vi "update_tab.vi"(8 "配置":T1 {"串口通信UI"."Format" items=["标准帧", "扩展帧"]; "串口通信UI"."Type" items=["数据帧", "远程帧"]; "串口通信UI"."ID" format="0x%x"; "串口通信UI"."Fliter" items=["接收所有类型"=1, "只接收标准帧"=2, "只接收扩展帧"=3]; "串口通信UI"."kBaudRate" items=["5k bps"=1, "10k bps"=2, "20k bps"=3, "40k bps"=4, "50k bps"=5, "80k bps"=6, "100k bps"=7, "125k bps"=8, "200k bps"=9, "250k bps"=10, "400k bps"=11, "500k bps"=12, "666k bps"=13, "800k bps"=14, "1000k bps"=15, "33.33k bps"=16, "66.66k bps"=17, "83.33k bps"=18]; "串口通信UI"."Mode" items=["正常工作", "仅侦听模式", "自测模式（环回）"]; "串口通信UI"."InitFlag" items=["使用界面设置参数"=1]; "串口通信UI"."AccMask" format="%08x"; "串口通信UI"."AccCode" format="%08x"; "串口通信UI"."Channel" items=["通道1", "通道2"]; "串口通信UI"."DevType" items=["USB-CAN"=3, "USB-CAN2"=4]; "安全报警UI"."操作 8" items=["产生报警信息（不发声），等待手动操作", "产生报警信息（发声），等待手动操作", "产生报警信息（不发声），自动刹车", "产生报警信息（发声），自动刹车", "产生报警信息（不发声），立即自动断电，开启泄放电阻", "产生报警信息（发声），立即自动断电，开启泄放电阻"]; "安全报警UI"."操作 7" items=["产生报警信息（不发声），等待手动操作", "产生报警信息（发声），等待手动操作", "产生报警信息（不发声），自动刹车", "产生报警信息（发声），自动刹车", "产生报警信息（不发声），立即自动断电，开启泄放电阻", "产生报警信息（发声），立即自动断电，开启泄放电阻"]; "安全报警UI"."操作 6" items=["产生报警信息（不发声），等待手动操作", "产生报警信息（发声），等待手动操作", "产生报警信息（不发声），自动刹车", "产生报警信息（发声），自动刹车", "产生报警信息（不发声），立即自动断电，开启泄放电阻", "产生报警信息（发声），立即自动断电，开启泄放电阻"]; "安全报警UI"."操作 5" items=["产生报警信息（不发声），等待手动操作", "产生报警信息（发声），等待手动操作", "产生报警信息（不发声），自动刹车", "产生报警信息（发声），自动刹车", "产生报警信息（不发声），立即自动断电，开启泄放电阻", "产生报警信息（发声），立即自动断电，开启泄放电阻"]; "安全报警UI"."操作 4" items=["产生报警信息（不发声），等待手动操作", "产生报警信息（发声），等待手动操作", "产生报警信息（不发声），自动刹车", "产生报警信息（发声），自动刹车", "产生报警信息（不发声），立即自动断电，开启泄放电阻", "产生报警信息（发声），立即自动断电，开启泄放电阻"]; "安全报警UI"."操作 3" items=["产生报警信息（不发声），等待手动操作", "产生报警信息（发声），等待手动操作", "产生报警信息（不发声），自动刹车", "产生报警信息（发声），自动刹车", "产生报警信息（不发声），立即自动断电，开启泄放电阻", "产生报警信息（发声），立即自动断电，开启泄放电阻"]; "安全报警UI"."操作 2" items=["产生报警信息（不发声），等待手动操作", "产生报警信息（发声），等待手动操作", "产生报警信息（不发声），自动刹车", "产生报警信息（发声），自动刹车", "产生报警信息（不发声），立即自动断电，开启泄放电阻", "产生报警信息（发声），立即自动断电，开启泄放电阻"]; "安全报警UI"."操作" items=["产生报警信息（不发声），等待手动操作", "产生报警信息（发声），等待手动操作", "产生报警信息（不发声），自动刹车", "产生报警信息（发声），自动刹车", "产生报警信息（不发声），立即自动断电，开启泄放电阻", "产生报警信息（发声），立即自动断电，开启泄放电阻"]}, 9 "簇":T22, 10 "结果字符串":string, 11 "是否是文件":bool) -> ()   [LabVIEW 2018, in "UI.lvlib"]
uses:
  UI.lvlib
  Settings/Settings.ctl
  Acquisition/Hardware Configuration.ctl
  Acquisition/Signal Type.ctl
  Acquisition/Acquisition.lvlib
  Settings/Settings.lvlib
panel:
  out "子字符串之前":string
  # "参数配置文件"
  # "输入数据文件"
  # "EHA电机"
  # "模拟电机"
  # "注：每次运行实验时销毁现有所有图像"
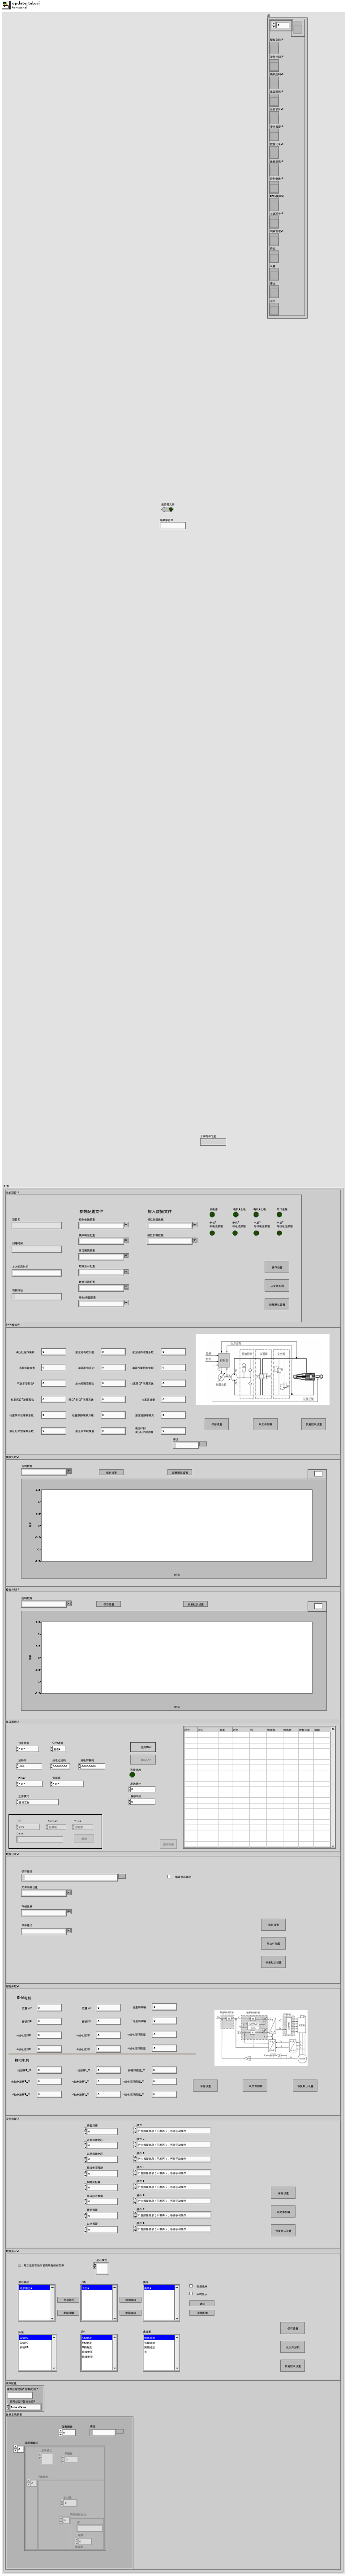
[diagram p1: front panel]
types:
  T1 = typedef "Settings.lvlib/Settings.ctl" = cluster{"当前项目UI":T2, "EHA模拟UI":T3, "模拟负载UI":T4, "模拟控制UI":T5, "串口通信UI":T6, "数据记录UI":T12, "控制参数UI":T13, "安全报警UI":T14, "数据显示UI":T15, "硬件配置":T16, "数据显示配置":T18}
  T2 = typedef "控件 5.ctl" = cluster{"控制参数配置":string, "模拟响应配置":string, "串口通信配置":string, "数据显示配置":string, "数据记录配置":string, "安全/报警配置":string, "模拟负载数据":string, "模拟加载数据":string, "总电源":bool, "电机1上电":bool, "电机2上电":bool, "串口连接":bool, "电机1\n相电流报警":bool, "电机2\n相电流报警":bool, "电机1\n母线电压报警":bool, "电机2\n母线电压报警":bool, "保存设置":bool, "从文件加载":bool, "恢复默认设置":bool, "路径":path, "项目路径":path, "项目名":string, "创建时间":string, "上次使用时间":string}
  T3 = typedef "EHA模拟UI.ctl" = cluster{"液压缸有效面积":dbl, "活塞初始位置":dbl, "气体多变系数k":dbl, "柱塞泵口2泄露系数":dbl, "柱塞泵粘性摩擦系数":dbl, "液压缸粘性摩擦系数":dbl, "液压缸有效长度":dbl, "油箱初始压力":dbl, "单向阀通流系数":dbl, "泵口1到口2泄露系数":dbl, "柱塞泵静摩擦力矩":dbl, "液压油体积模量":dbl, "保存设置":bool, "从文件加载":bool, "恢复默认设置":bool, "路径":path, "液压缸内泄露系数":dbl, "油箱气囊初始体积":dbl, "柱塞泵口1泄露系数":dbl, "柱塞泵排量":dbl, "液压缸静摩擦力":dbl, "液压杆到\n液压缸的总质量":dbl}
  T4 = typedef "控件 9.ctl" = cluster{"负载数据":string, "负载数据 2":waveform(dbl)[], "保存设置":bool, "恢复默认设置":bool}
  T5 = typedef "控件 7.ctl" = cluster{"控制数据":string, "负载数据 2":waveform(dbl)[], "保存设置":bool, "恢复默认设置":bool}
  T6 = typedef "控件 6.ctl" = cluster{"DevType":T7, "Channel":T8, "AccCode":u32, "AccMask":u32, "InitFlag":T9, "Mode":T10, "kBaudRate":u8, "Fliter":T11, "Open":bool, "Close":bool, "连接状态":bool, "SendCnt":u32, "RecvCnt":u32, "Send":bool, "ID":u32, "Data":string, "Type":u8, "Format":u8, "Clear":bool, "list":i32, "路径":path}
  T7 = typedef "ControlCAN.lvlib/DevType.ctl" = u32
  T8 = typedef "ControlCAN.lvlib/CAN Channel.ctl" = u32
  T9 = typedef "ControlCAN.lvlib/InitFlag.ctl" = u32
  T10 = typedef "ControlCAN.lvlib/Mode.ctl" = u8
  T11 = typedef "ControlCAN.lvlib/Fliter.ctl" = u8
  T12 = typedef "控件 3.ctl" = cluster{"保存路径":path, "文件命名设置":string, "存储数据":string, "保存格式":string, "复选框":bool, "保存设置":bool, "从文件加载":bool, "恢复默认设置":bool, "路径":path, "TDMS文件引用":refnum<k34>}
  T13 = typedef "控件 1.ctl" = cluster{"d轴电流环P_M":dbl, "转速环P":dbl, "q轴电流环P":dbl, "d轴电流环P":dbl, "转矩环P_M":dbl, "去轴电流环P_M":dbl, "转速环I":dbl, "q轴电流环I":dbl, "d轴电流环I":dbl, "转矩环I_M":dbl, "q轴电流环I_M":dbl, "d轴电流环I_M":dbl, "保存设置":bool, "从文件加载":bool, "恢复默认设置":bool, "路径":path, "位置环P":dbl, "位置环I":dbl, "转速环限幅":dbl, "q轴电流环限幅":dbl, "d轴电流环限幅":dbl, "位置环限幅":dbl, "转矩环限幅_M":dbl, "q轴电流环限幅_M":dbl, "d轴电流环限幅_M":dbl}
  T14 = typedef "控件 4.ctl" = cluster{"报警扭矩":dbl, "过低母线电压":dbl, "过高母线电压":dbl, "母线电流限制":dbl, "相电流报警":dbl, "串口超时报警":dbl, "转速报警":dbl, "过热报警":dbl, "操作":u16, "操作 2":u16, "操作 3":u16, "操作 4":u16, "操作 5":u16, "操作 6":u16, "操作 7":u16, "操作 8":u16, "保存设置":bool, "从文件加载":bool, "恢复默认设置":bool, "路径":path}
  T15 = typedef "控件 2.ctl" = cluster{"保存设置":bool, "从文件加载":bool, "恢复默认设置":bool, "实验":i32, "波形输出":i32, "组件":i32, "曲线":i32, "滤波器":i32, "删除曲线":bool, "清理图像":bool, "添加曲线":bool, "数据选点":bool, "确定按钮":bool, "实时显示":bool, "子图":i32, "显示模式":u16, "路径":path, "删除图像":bool, "创建新图":bool}
  T16 = typedef "Acquisition.lvlib/Hardware Configuration.ctl" = cluster{"硬件引用句柄<替换此项>":string, "信号类型<替换该项>":T17}
  T17 = typedef "Acquisition.lvlib/Signal Type.ctl" = enum16{"Sine Wave", "Square with Noise"}
  T18 = typedef "波形图簇.ctl" = cluster{"波形图数":u32, "波形图数组":T19[], "路径":path}
  T19 = typedef "波形图.ctl" = cluster{"显示模式":u16, "子图数":u32, "子图数组":T20[]}
  T20 = typedef "子图.ctl" = cluster{"子图所有曲线":T21[], "曲线数":u32}
  T21 = typedef "曲线簇.ctl" = cluster{"源":string, "组件":u32, "滤波器":u32}
  T22 = typedef "引用簇.ctl" = cluster{"数组":refnum<vi>[], "模拟负载UI":refnum<vi>, "波形控制UI":refnum<vi>, "模拟控制UI":refnum<vi>, "串口通信UI":refnum<vi>, "当前项目UI":refnum<vi>, "安全报警UI":refnum<vi>, "数据记录UI":refnum<vi>, "数据显示UI":refnum<vi>, "控制参数UI":refnum<vi>, "EHA模拟UI":refnum<vi>, "主选项卡UI":refnum<vi>, "项目管理UI":refnum<vi>, "开始":refnum<vi>, "设置":refnum<vi>, "停止":refnum<vi>, "退出":refnum<vi>}
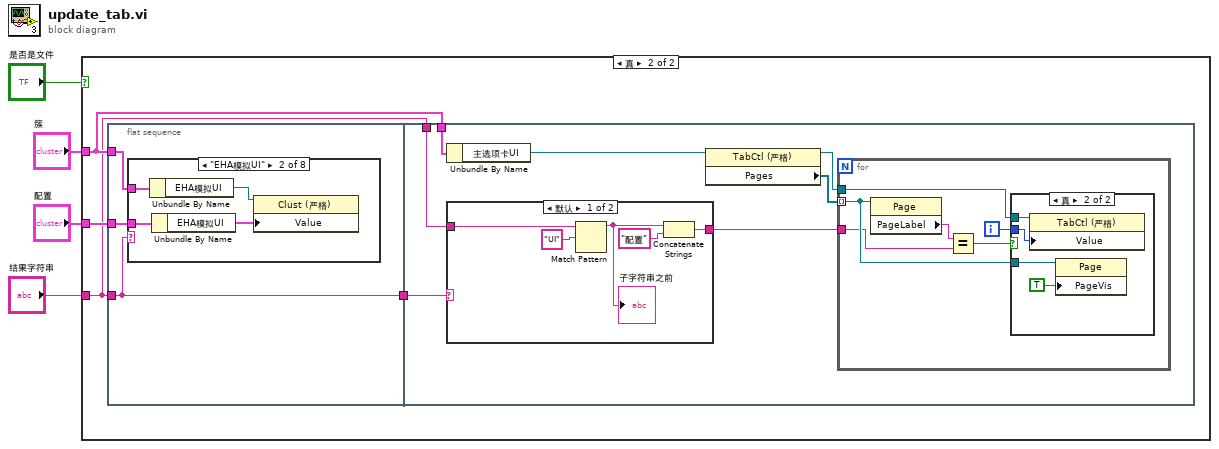
[diagram p0: block diagram]
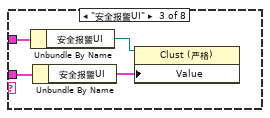
[diagram p4: hidden frame]
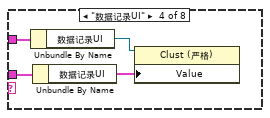
[diagram p5: hidden frame]
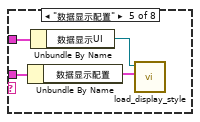
[diagram p6: hidden frame]
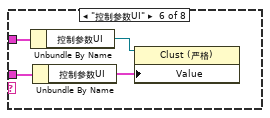
[diagram p7: hidden frame]
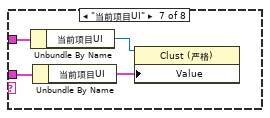
[diagram p8: hidden frame]
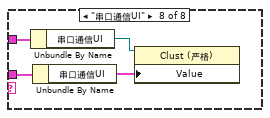
[diagram p9: hidden frame]
diagram:
  n1 = case shown="真" "是否是文件" {
    tunnel: "结果字符串" -> [_ w5]
    tunnel: "簇" -> [_ w8]
    tunnel: "配置" -> [_ w7]
    frame False {
    }
    frame True {
      n2 = flat-sequence {
        tunnel: w5 -> [w9]
        tunnel: w8 -> [w11]
        tunnel: w7 -> [w10]
        tunnel: [w9] -> w6
        tunnel: w8 -> [w43]
        tunnel: w6 -> [w42]
        tunnel: w5 -> [w41]
        frame #0 {
          n3 = case shown="\"EHA模拟UI\"" w9 {
            tunnel: w11 -> [_ w12 w19 w23 w27 w31 w35 w39]
            tunnel: w10 -> [_ w13 w18 w22 w26 w29 w34 w38]
            frame Default {
            }
            frame "EHA模拟UI" {
              n4 = Unbundle By Name(w12) -> ("EHA模拟UI"=w15:refnum<vi>)
              n5 = Unbundle By Name(w13) -> ("EHA模拟UI"=w14:T3)
              n6 = property class="Clust (严格)"(reference=w15, "Value"=w14) -> ()  [unwired: 1 in, 2 out]
            }
            frame "安全报警UI" {
              n7 = Unbundle By Name(w19) -> ("安全报警UI"=w17:refnum<vi>)
              n8 = Unbundle By Name(w18) -> ("安全报警UI"=w16:T14)
              n9 = property class="Clust (严格)"(reference=w17, "Value"=w16) -> ()  [unwired: 1 in, 2 out]
            }
            frame "数据记录UI" {
              n10 = Unbundle By Name(w23) -> ("数据记录UI"=w21:refnum<vi>)
              n11 = Unbundle By Name(w22) -> ("数据记录UI"=w20:T12)
              n12 = property class="Clust (严格)"(reference=w21, "Value"=w20) -> ()  [unwired: 1 in, 2 out]
            }
            frame "数据显示配置" {
              n13 = Unbundle By Name(w26) -> ("数据显示配置"=w25:T18)
              n14 = Unbundle By Name(w27) -> ("数据显示UI"=w24:refnum<vi>)
              n15 = call "load_display_style.vi"("数据显示配置"=w25, "Cluster输入"=w24) -> ()  [unwired: 10 in]
            }
            frame "控制参数UI" {
              n16 = Unbundle By Name(w31) -> ("控制参数UI"=w30:refnum<vi>)
              n17 = Unbundle By Name(w29) -> ("控制参数UI"=w28:T13)
              n18 = property class="Clust (严格)"(reference=w30, "Value"=w28) -> ()  [unwired: 1 in, 2 out]
            }
            frame "当前项目UI" {
              n19 = Unbundle By Name(w35) -> ("当前项目UI"=w33:refnum<vi>)
              n20 = Unbundle By Name(w34) -> ("当前项目UI"=w32:T2)
              n21 = property class="Clust (严格)"(reference=w33, "Value"=w32) -> ()  [unwired: 1 in, 2 out]
            }
            frame "串口通信UI" {
              n22 = Unbundle By Name(w39) -> ("串口通信UI"=w37:refnum<vi>)
              n23 = Unbundle By Name(w38) -> ("串口通信UI"=w36:T6)
              n24 = property class="Clust (严格)"(reference=w37, "Value"=w36) -> ()  [unwired: 1 in, 2 out]
            }
          }
        }
        frame #1 {
          n25 = Unbundle By Name(w43) -> ("主选项卡UI"=w44:refnum<vi>)
          n26 = case shown="默认" w42 {
            tunnel: w41 -> [w51 w52]
            tunnel: [w47 w52] -> w40
            frame Default {
              n27 = Match Pattern(string=w51, regular expression="UI" ("正则表达式")) -> (before substring=w49:string)  [unwired: 1 in, 3 out]
              "子字符串之前" <- w49
              n28 = Concatenate Strings(w49, "配置" ("字符串")) -> (w47:string)
            }
            frame "数据显示配置" {
            }
          }
          n29 = property class="TabCtl (严格)"(reference=w44) -> (reference out=w45:refnum<vi>, "Pages"=w46:refnum<vi>[])  [unwired: 1 in, 1 out]
          n30 = for {
            tunnel: w46 -> [w58] mode=indexing
            tunnel: w40 -> [w55]
            tunnel: w45 -> [w54]
            i -> [w53]
            n31 = property class="Page"(reference=w58) -> ("PageLabel"=w56:string)  [unwired: 1 in, 2 out]
            n32 = Equal?(x=w56, y=w55) -> (x = y?=w57:bool)
            n33 = case shown="真" w57 {
              tunnel: w58 -> [_ w62]
              tunnel: w54 -> [_ w60]
              tunnel: w53 -> [_ w59]
              frame False {
              }
              frame True {
                n34 = property class="TabCtl (严格)"(reference=w60, "Value"=w59) -> ()  [unwired: 1 in, 2 out]
                n35 = property class="Page"(reference=w62, "PageVis"=TRUE ("选项卡可见")) -> ()  [unwired: 1 in, 2 out]
              }
            }
          }
        }
      }
    }
  }
